vi "Dispose Report.vi"(0 "report in":refnum<class "ooCalc.lvclass">, 5 "wait until printing completed? (T)":bool=TRUE, 9 "save changes? (F)":bool, 11 "error in (no error)":errorcluster, 12 "close report? (T)":bool=TRUE) -> (15 "error out":errorcluster)   [LabVIEW 2009, in "ooCalc.lvclass"]
doc: "Closes the report and releases its interface, which saves memory."
uses:
  ooCalc.lvclass
  ooCalc.lvclass/ooCalc.ctl
  C:/Projets/LAVAG/OpenOfficeRGT/AODL/DLLs/AODL.dll
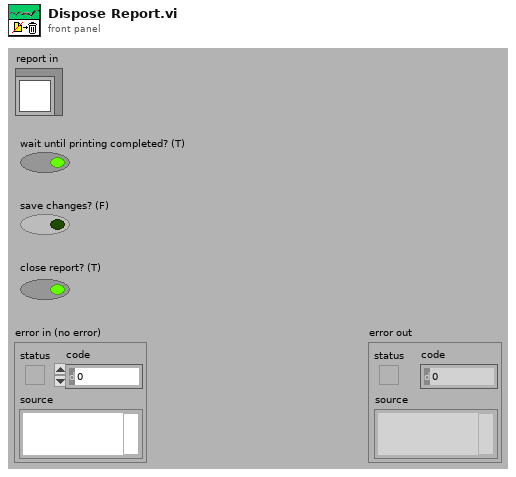
[diagram p1: front panel]
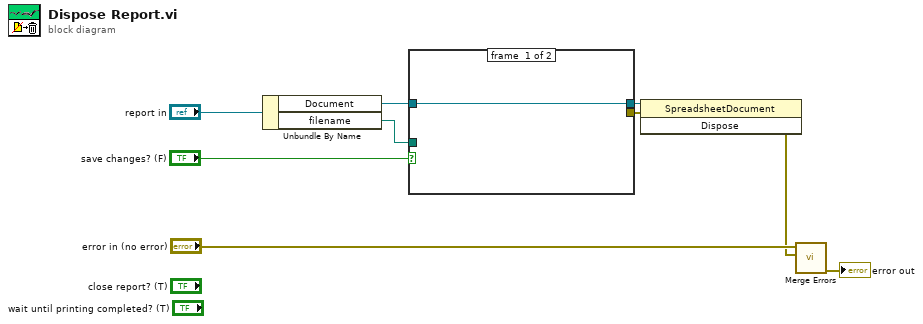
[diagram p0: block diagram]
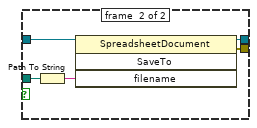
[diagram p2: hidden frame]
diagram:
  n1 = Unbundle By Name("report in") -> ("Document"=w7:refnum<k24>, "filename"=w6:path)
  n2 = case shown="True" "save changes? (F)" {
    tunnel: w7 -> [w10 w15]
    tunnel: [w10 w14] -> w5
    tunnel: w6 -> [_ w13]
    tunnel: [_ w11] -> w4
    frame #0 {
    }
    frame #1 {
      n3 = Path To String(path=w13) -> (string=w12:string)
      n4 = invoke class="SpreadsheetDocument" method="SaveTo"(reference=w15, "filename"=w12) -> (reference out=w14:refnum<k24>, error out=w11:errorcluster)  [unwired: 2 in, 2 out]
    }
  }
  n5 = invoke class="SpreadsheetDocument" method="Dispose"(reference=w5, error in=w4) -> (error out=w2:errorcluster)  [unwired: 1 in, 2 out]
  n6 = call <vilib>:"Merge Errors.vi"("error in 2 (no error)"=w2, "error in 1 (no error)"="error in (no error)") -> ("error out"=→"error out":errorcluster)  [unwired: 5 in]
